vi "close.vi"(8 "error in":errorcluster, 11 "deviceHandle":i32) -> (0 "error out":errorcluster)   [LabVIEW 2016]
uses:
  DLLHandler/Release/LabVIEWJSON.dll
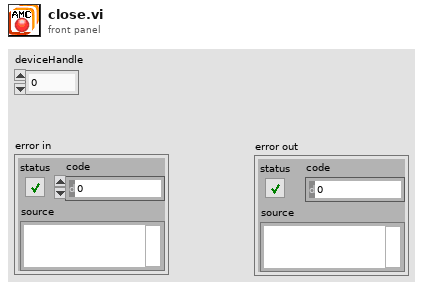
[diagram p1: front panel]
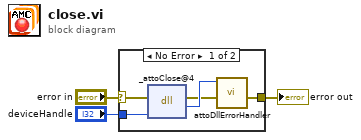
[diagram p0: block diagram]
diagram:
  n1 = case shown="No Error" "error in" {
    selector: "error in" -> [w5 w9]
    tunnel: "deviceHandle" -> [w8 _]
    tunnel: [w4 w9] -> w1
    frame No Error {
      n2 = dll-call lib="C:/Users/schieda/OneDrive - WITTENSTEIN SE/Desktop/LabVIEW/API_Autogen_v1.3_DSc/generatedAPIs/AMC_VIs_DLL (for older LV Versions only)/DLLHandler/Release/LabVIEWJSON.dll" fn="_attoClose@4"(error in=w5, "deviceHandle"=w8) -> (error out=w6:errorcluster, "rc"=w7:i32)  [unwired: 3 in, 1 out]
      n3 = call "attoDllErrorHandler.vi"("error in"=w6, "rc"=w7) -> ("error out"=w4:errorcluster)  [unwired: 9 in]
    }
    frame Error {
    }
  }
  "error out" <- w1
